vi "swerve_forwards_kinematics.vi"() -> (0 "v_x":dbl(slide) scale=-1.0..1.0, 2 "v_y":dbl(slide) scale=-1.0..1.0, 4 "omega":dbl(slide) scale=-1.0..1.0, 20 "v_0":dbl, 21 "theta_0":dbl, 22 "v_1":dbl, 23 "theta_1":dbl, 24 "v_2":dbl, 25 "theta_2":dbl, 26 "v_3":dbl, 27 "theta_3":dbl)   [LabVIEW 2020]
uses:
  <vilib>/Analysis/Matrix/Datatypes/RealMatrix.ctl
  <vilib>/Analysis/_algsub.llb/Real PseudoInverse Matrix.vi
  <vilib>/Analysis/Matrix/Numeric/Conversions/Array To Matrix - RA2.vi
  <vilib>/Analysis/Matrix/Numeric/Multiply/Multiply - RM,RM.vi
  <vilib>/Analysis/Matrix/NI_Matrix.lvlib
  <vilib>/Analysis/NI_AALPro.lvlib
panel:
  in  "Input Vector":T1
  out "Output Vector":T1
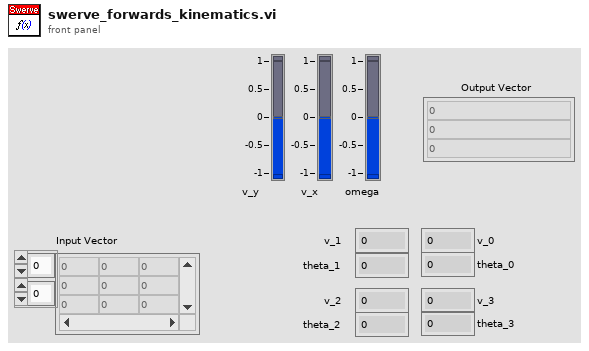
[diagram p1: front panel]
types:
  T1 = typedef "NI_Matrix.lvlib/RealMatrix.ctl" = dbl[][]
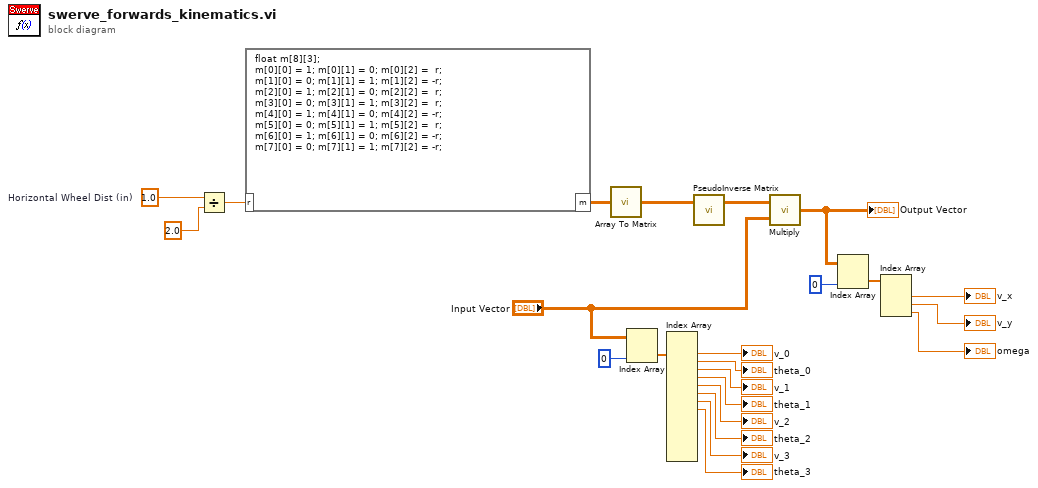
[diagram p0: block diagram]
diagram:
  w13 = 1.0  # Horizontal Wheel Dist (in)
  n1 = Divide(x=w13, y=2.0) -> (x/y=w23:dbl)
  n2 = formula code="float m[8][3];\nm[0][0] = 1; m[0][1] = 0; m[0][2] =  r;\nm[1][0] = 0; m[1][1] = 1; m[1][2] = -r;\nm[2][0] = 1; m[2][1] = 0; m[2][2] =  r;\nm[3][0] = 0; m[3][1] = 1; m[3][2] =  r;\nm[4][0] = 1; m[4][1] = 0; m[4][2] = -r;\nm[5][0] = 0; m[5][1] = 1; m[5][2] =  r;\nm[6][0] = 1; m[6][1] = 0; m[6][2] = -r;\nm[7][0] = 0; m[7][1] = 1; m[7][2] = -r;"("r"=w23) -> ("m"=w22:dbl[][])
  n3 = call-poly <vilib>:"Array To Matrix.vi"("Real 2D Array"=w22) -> ("Real Matrix"=w21:T1)
  n4 = Index Array(array="Input Vector", index (col)=0 ("disabled index (col)")) -> (element=w10:dbl[])  [unwired: 1 in]
  n5 = Index Array(array=w10) -> (element #1=→"v_0":dbl, element #2=→"theta_0":dbl, element #3=→"v_1":dbl, element #4=→"theta_1":dbl, element #5=→"v_2":dbl, element #6=→"theta_2":dbl, element #7=→"v_3":dbl, element #8=→"theta_3":dbl)  [unwired: 14 in, 6 out]
  n6 = call-poly <vilib>:"PseudoInverse Matrix.vi"("Input Matrix"=w21) -> ("PseudoInverse Matrix"=w20:T1)  [unwired: 1 in, 1 out]
  n7 = call-poly <vilib>:"Multiply.vi"("Real Matrix B"="Input Vector", "Real Matrix A"=w20) -> ("A * B"=w19:T1)
  "Output Vector" <- w19
  n8 = Index Array(array=w19, index (col)=0 ("disabled index (col)")) -> (element=w17:dbl[])  [unwired: 1 in]
  n9 = Index Array(array=w17) -> (element #1=→"v_x":dbl, element #2=→"v_y":dbl, element #3=→"omega":dbl)  [unwired: 3 in]
